vi "Get Reentrancy State.vi"(8 "error in":errorcluster, 11 "File Info in":T1) -> (0 "error out":errorcluster, 3 "File Info out":T1)   [LabVIEW 2020, in "Peer Review.lvclass"]
uses:
  Peer Review.lvclass
  TypeDefs/File Info.ctl
  TypeDefs/File State.ctl
  TypeDefs/VI Type.ctl
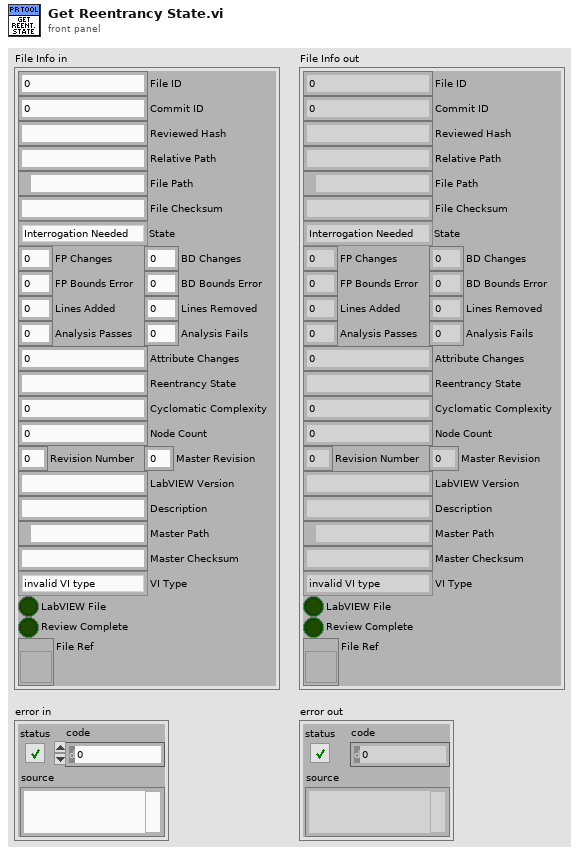
[diagram p1: front panel]
types:
  T1 = typedef "Peer Review.lvclass/File Info.ctl" = cluster{"File ID":i32, "Commit ID":i32, "Reviewed Hash":string, "Relative Path":string, "File Path":path, "File Checksum":string, "State":T2, "FP Changes":i32, "BD Changes":i32, "FP Bounds Error":dbl, "BD Bounds Error":dbl, "Lines Added":i32, "Lines Removed":i32, "Analysis Passes":i32, "Analysis Fails":i32, "Attribute Changes":i32, "Reentrancy State":string, "Cyclomatic Complexity":i32, "Node Count":i32, "Revision Number":u32, "LabVIEW Version":string, "Description":string, "Master Path":path, "Master Checksum":string, "VI Type":T3, "LabVIEW File":bool, "Review Complete":bool, "File Ref":refnum<vi>, "Master Revision":u32}
  T2 = typedef "Peer Review.lvclass/File State.ctl" = enum16{"Interrogation Needed", "Modified", "Deleted", "Added", "Matches Previous", "No Changes", "Moved", "Empty File"}
  T3 = typedef "Peer Review.lvclass/VI Type.ctl" = enum32{"invalid VI type", "Standard VI", "Control VI", "Global VI", "Polymorphic VI", "Configuration VI", "SubSystem", "Facade VI", "Method VI", "Statechart Diagram VI"}
  T4 = enum16{"Share clones between instances", "Preallocate clone for each instance"}
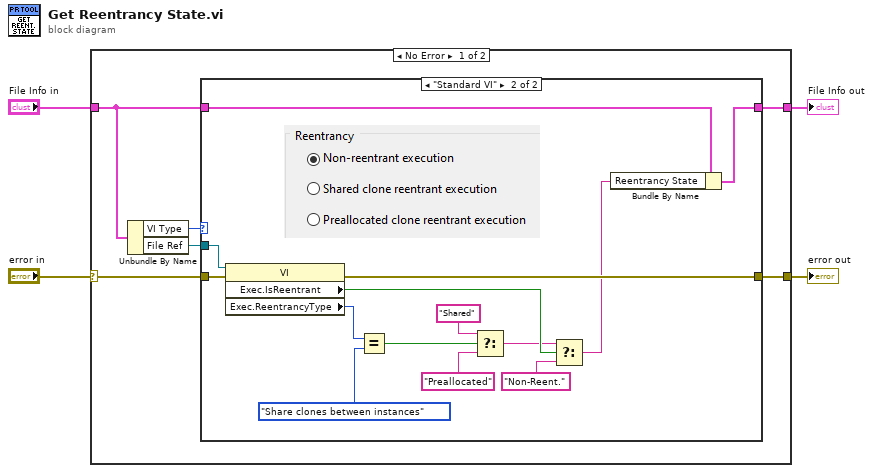
[diagram p0: block diagram]
diagram:
  n1 = case shown="No Error" "error in" {
    selector: "error in" -> [w5 w28]
    tunnel: [w10 w28] -> w4
    tunnel: "File Info in" -> [w8 w27]
    tunnel: [w9 w27] -> w1
    frame No Error {
      n2 = Unbundle By Name(w8) -> ("VI Type"=w7:T3, "File Ref"=w6:refnum<vi>)
      n3 = case shown="\"Standard VI\"" w7 {
        tunnel: [w11 w14] -> w10
        tunnel: w5 -> [w11 w26]
        tunnel: w6 -> [_ w25]
        tunnel: w8 -> [w12 w16]
        tunnel: [w12 w15] -> w9
        frame Default {
        }
        frame "Standard VI" {
          n4 = property on="Property Node" class="VI"(reference=w25, error in=w26) -> (error out=w14:errorcluster, "Exec.IsReentrant"=w21:bool, "Exec.ReentrancyType"=w24:T4)  [unwired: 1 out]
          n5 = Equal?(x=w24, y=T4."Share clones between instances") -> (x = y?=w22:bool)
          n6 = Select(t="Shared", s=w22, f="Preallocated") -> (s? t:f=w20:string)
          n7 = Select(t=w20, s=w21, f="Non-Reent.") -> (s? t:f=w13:string)
          n8 = Bundle By Name(cluster=w16, "Reentrancy State"=w13) -> (w15:T1)
        }
      }
    }
    frame Error {
    }
  }
  "error out" <- w4
  "File Info out" <- w1
